vi "IsSourceInCompliance.vi"(7 "SMU":T1, 8 "Error In":errorcluster, 11 "Kiethley 2602 In":refnum<visa-resource-name>) -> (0 "Error Out":errorcluster, 2 "Compliance?":bool, 3 "Keithley 2602 Out":refnum<visa-resource-name>)   [LabVIEW 2012, in "Keithley-2602.lvlib"]
uses:
  Keithley-2602.lvlib
  Controls/SMU.ctl
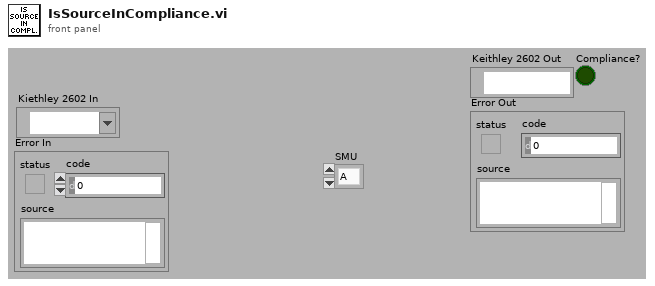
[diagram p1: front panel]
types:
  T1 = typedef "Keithley-2602.lvlib/SMU.ctl" = enum16{"A", "B"}
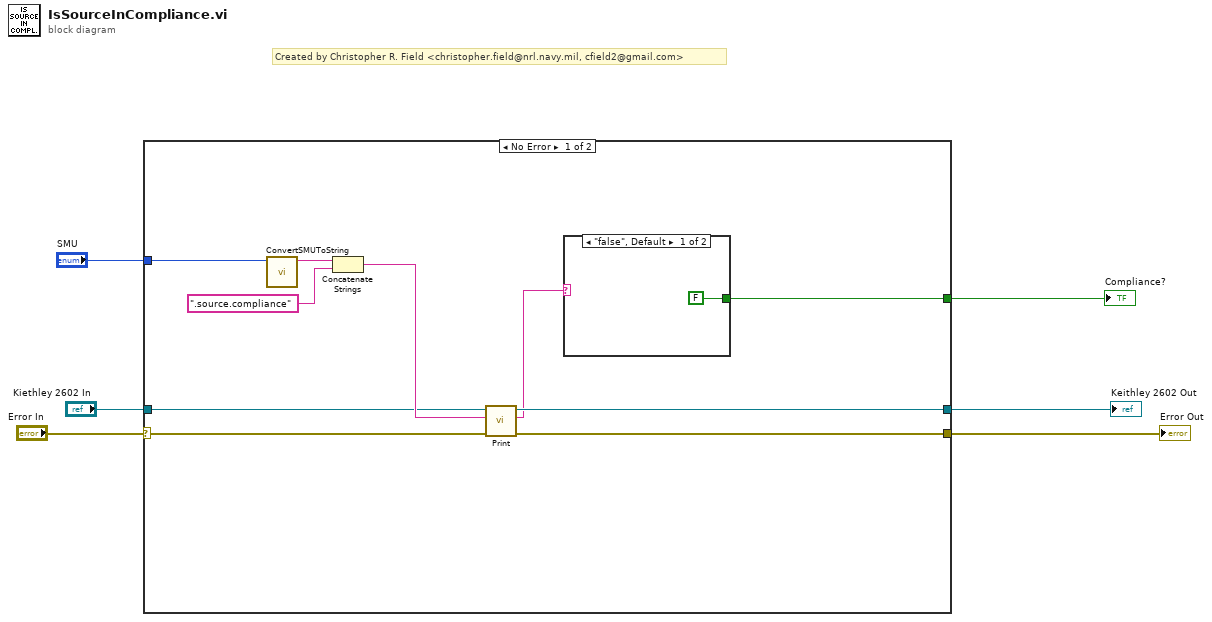
[diagram p0: block diagram]
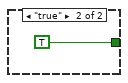
[diagram p2: hidden frame]
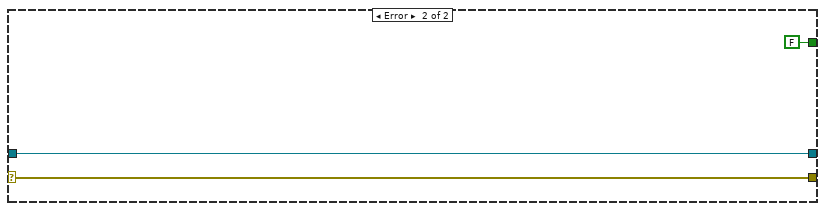
[diagram p3: hidden frame]
diagram:
  # "Created by Christopher R. Field <christopher.field@nrl.navy.mil, cfield2@gmail.com>"
  n1 = case shown="No Error" "Error In" {
    selector: "Error In" -> [w7 w21]
    tunnel: "Kiethley 2602 In" -> [w13 w20]
    tunnel: [w12 w20] -> w5
    tunnel: [w11 w21] -> w4
    tunnel: [w9 FALSE] -> w3
    tunnel: "SMU" -> [w8 _]
    frame No Error {
      n2 = call "ConvertSMUToString.vi"("SMU"=w8) -> ("Channel"=w16:string)  [unwired: 10 in]
      n3 = Concatenate Strings(w16, ".source.compliance") -> (w14:string)
      n4 = call "Print.vi"("Error In"=w7, "Attribute"=w14, "Kiethley 2602 In"=w13) -> ("Error Out"=w11:errorcluster, "Output"=w10:string, "Keithley 2602 Out"=w12:refnum<visa-resource-name>)  [unwired: 6 in]
      n5 = case shown="\"false\", Default" w10 {
        tunnel: [FALSE TRUE] -> w9
        frame "false", Default {
        }
        frame "true" {
        }
      }
    }
    frame Error {
    }
  }
  "Keithley 2602 Out" <- w5
  "Error Out" <- w4
  "Compliance?" <- w3
